vi "piezoGetPosFromFrameCount.vi"(1 "optimize (T)":bool=TRUE, 2 "frame counts":i32[](array[numeric])) -> (0 "piezo pos":dbl[](array[numeric]))   [LabVIEW 2017]
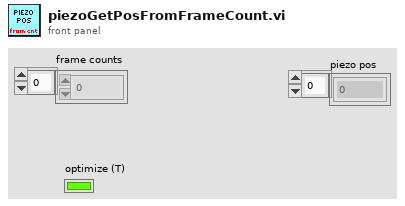
[diagram p1: front panel]
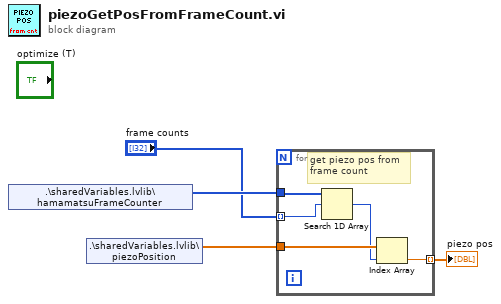
[diagram p0: block diagram]
diagram:
  n1 = shared-variable ".\\sharedVariables.lvlib\\hamamatsuFrameCounter"() -> (w4:u32[])  [unwired: 1 in, 1 out]
  n2 = shared-variable ".\\sharedVariables.lvlib\\piezoPosition"() -> (w3:dbl[])  [unwired: 1 in, 1 out]
  n3 = for {
    tunnel: "frame counts" -> [w8] mode=indexing
    tunnel: w4 -> [w9]
    tunnel: w3 -> [w7]
    tunnel: [w5] -> w1 mode=indexing
    # "get piezo pos from\nframe count"
    n4 = Search 1D Array(1D array=w9, element=w8) -> (index of element=w6:i32)  [unwired: 1 in]
    n5 = Index Array(array=w7, index=w6) -> (element=w5:dbl)
  }
  "piezo pos" <- w1
